vi "NotifyIcon - Create.vi"(8 "error in":errorcluster, 10 "Context Menu (optional)":string[][](array[string]), 11 "Icon File Path":path=path "C:/Program Files/National Instruments/LabVIEW 2009/applibs/lvapp.ico") -> (0 "error out":errorcluster, 3 "NotifyIcon reference":refnum<k24>)   [LabVIEW 2020]
doc: "Creates an Icon, specified by <b>Icon File Path</b>, in the notification area of the Windows task bar.\n\n<b>Context Menu (optional)</b> will create a pop-up menu that will be shown when the Icon is right-clicked."
uses:
  System.Windows.Forms
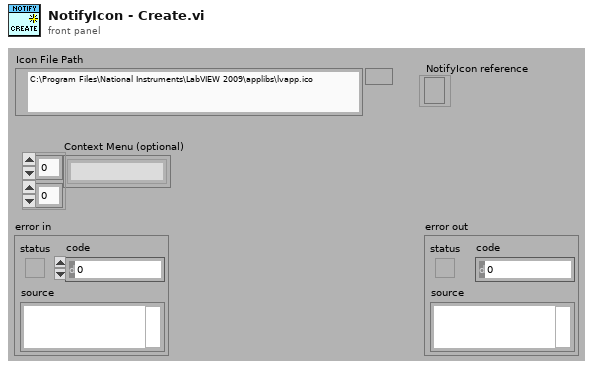
[diagram p1: front panel]
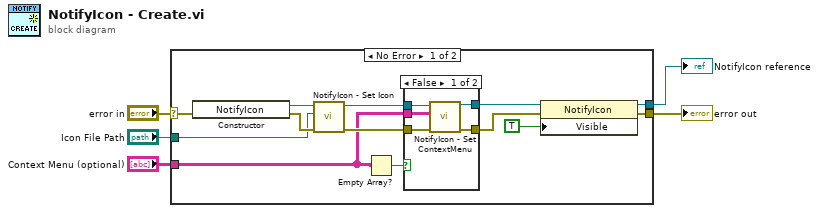
[diagram p0: block diagram]
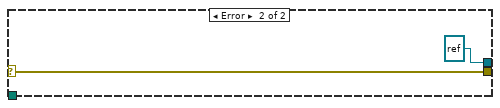
[diagram p3: hidden frame]
diagram:
  n1 = case shown="No Error" "error in" {
    selector: "error in" -> [w6 w26]
    tunnel: [w18 w26] -> w5
    tunnel: [w17 refnum<k24> refnum ("NotifyIcon reference out")] -> w4
    tunnel: "Icon File Path" -> [w14 _]
    tunnel: "Context Menu (optional)" -> [w8 _]
    frame No Error {
      n2 = constructor class="NotifyIcon"(error in=w6) -> (reference out=w16:refnum<k24>, error out=w15:errorcluster)  [unwired: 2 in, 1 out]
      n3 = call "NotifyIcon - Set Icon.vi"("error in"=w15, "Icon File Path"=w14, "NotifyIcon reference in"=w16) -> ("error out"=w11:errorcluster, "NotifyIcon reference out"=w12:refnum<k24>)  [unwired: 7 in]
      n4 = Empty Array?(array=w8) -> (empty?=w7:bool)
      n5 = case shown="False" w7 {
        tunnel: w12 -> [w23 w24]
        tunnel: w11 -> [w22 w25]
        tunnel: [w21 w25] -> w10
        tunnel: [w20 w24] -> w9
        tunnel: w8 -> [w19 _]
        frame False {
          n6 = call "NotifyIcon - Set ContextMenu.vi"("error in"=w22, "Context Menu"=w19, "NotifyIcon reference in"=w23) -> ("error out"=w21:errorcluster, "NotifyIcon reference out"=w20:refnum<k24>)  [unwired: 7 in]
        }
        frame True {
        }
      }
      n7 = property class="NotifyIcon"(reference=w9, error in=w10, "Visible"=TRUE) -> (reference out=w17:refnum<k24>, error out=w18:errorcluster)
    }
    frame Error {
    }
  }
  "error out" <- w5
  "NotifyIcon reference" <- w4
